vi "Append Multiple Waveforms.vi"(8 "error in (no error)":errorcluster, 10 "Waveform B []":waveform(dbl)[](array[waveform]), 11 "Waveforrm A []":waveform(dbl)[](array[waveform])) -> (0 "error out":errorcluster, 3 "Waveform out []":waveform(dbl)[](array[waveform]))   [LabVIEW 2019, in "Instrument.Lockin.lvlib" / "Instrument.DAQ.lvclass"]
uses:
  Instrument.DAQ.lvclass
  <vilib>/Waveform/WDTOps.llb/WDT Append Waveforms DBL.vi
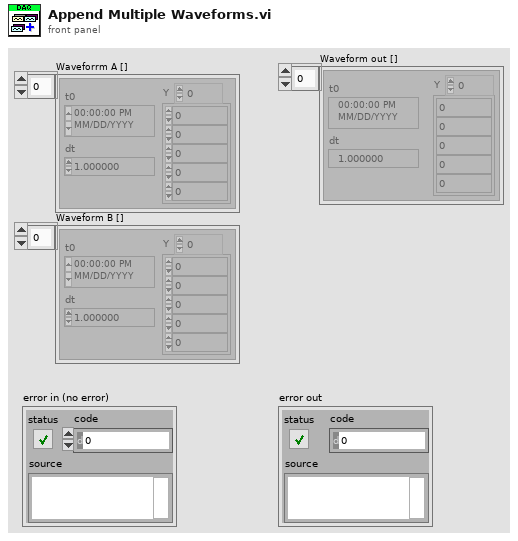
[diagram p1: front panel]
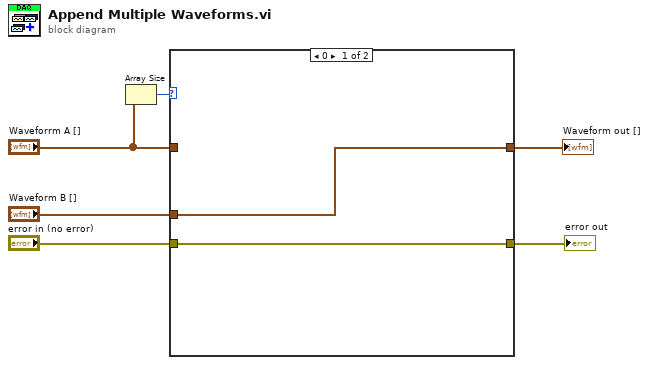
[diagram p0: block diagram]
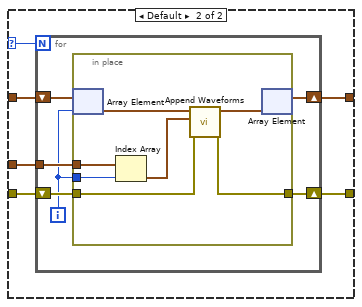
[diagram p2: hidden frame]
diagram:
  n1 = Array Size(array="Waveforrm A []") -> (size(s)=w2:i32)
  n2 = case shown="0" w2 {
    selector: w2 -> [_ w9]
    tunnel: [w8 w14] -> w6
    tunnel: "error in (no error)" -> [w7 w13]
    tunnel: "Waveforrm A []" -> [_ w12]
    tunnel: "Waveform B []" -> [w8 w11]
    tunnel: [w7 w10] -> w3
    frame 0 {
    }
    frame Default {
      n3 = for {
        N: w9 -> [_]
        tunnel: w11 -> [w18]
        shift-right: [w16] -> w14
        shift-left: w12 -> [w17]
        shift-right: [w19] -> w10
        shift-left: w13 -> [w20]
        i -> [w15]
        n4 = in-place {
          in-place-border: w20 -> [w22]
          in-place-border: [w21] -> w19
          in-place-border: w18 -> [w27]
          in-place-border: w15 -> [w25]
          n5 = in-place-array #1(w17, w15) -> (w24:waveform(dbl))
          n6 = Index Array(array=w27, index=w25) -> (element=w26:waveform(dbl))
          n7 = call-poly <vilib>:"Append Waveforms.vi"("error in (no error)"=w22, "waveform B"=w26, "waveform A"=w24) -> ("error out"=w21:errorcluster, "waveform out"=w23:waveform(dbl))  [unwired: 7 in]
          n8 = in-place-array #1(w23) -> (w16:waveform(dbl)[])  [unwired: 1 out]
        }
      }
    }
  }
  "error out" <- w3
  "Waveform out []" <- w6
